vi "n3.vi"(6 "Analysis":u8, 7 "beta":dbl, 8 "m":dbl, 9 "P":dbl, 10 "Segmentation A":dbl[](array[numeric]), 11 "Segmentation B":dbl[](array[numeric])) -> (1 "X2_tau":dbl[][](array[numeric]), 2 "X2_i":dbl[][](array[numeric]))   [LabVIEW 2015]
uses:
  <vilib>/Analysis/baseanly.llb/Mean (DBL).vi
  <vilib>/Analysis/NI_AALBase.lvlib
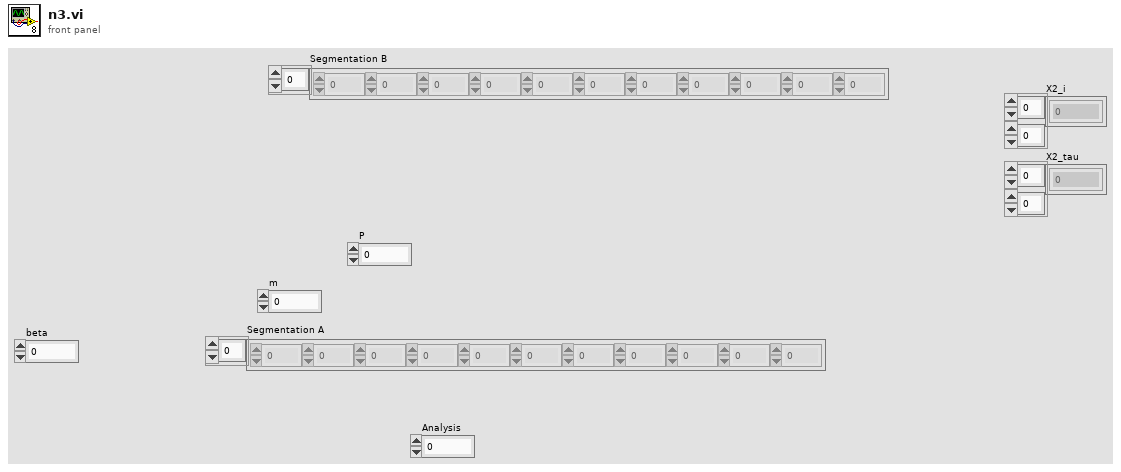
[diagram p1: front panel]
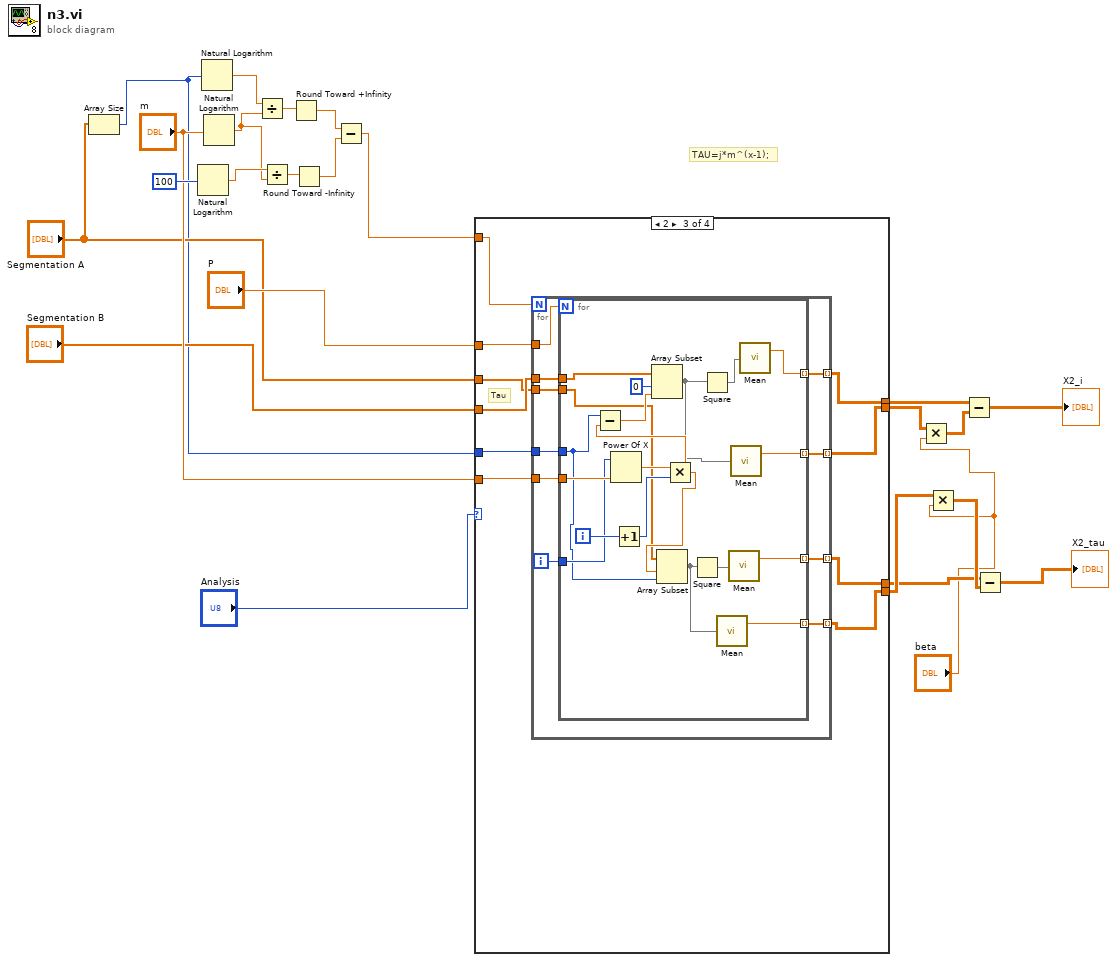
[diagram p0: block diagram]
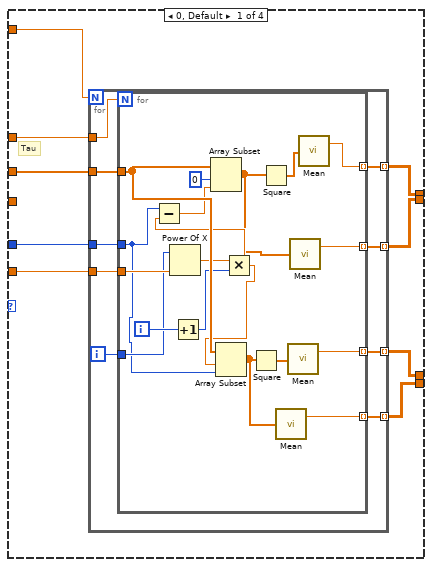
[diagram p2: hidden frame]
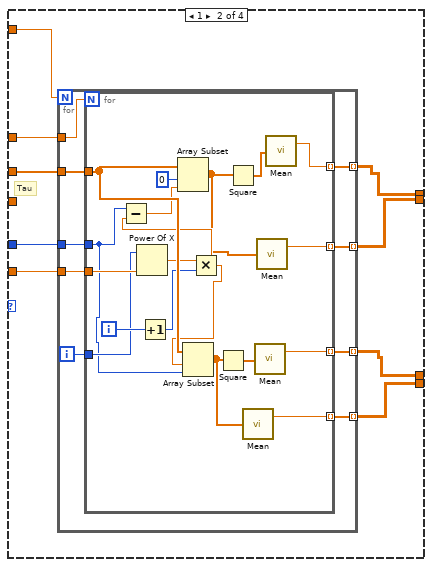
[diagram p3: hidden frame]
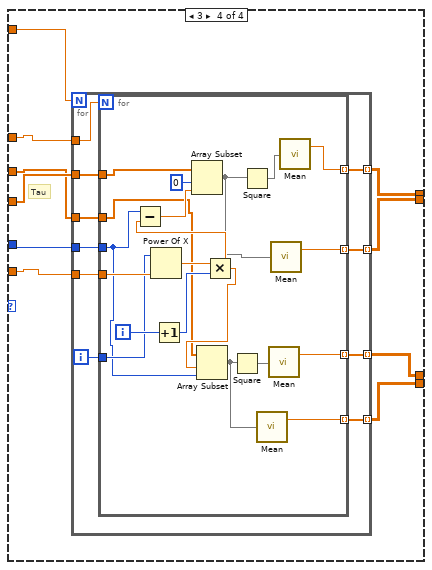
[diagram p4: hidden frame]
diagram:
  # "TAU=j*m^(x-1);"
  n1 = Array Size(array="Segmentation A") -> (size(s)=w4:i32)
  n2 = Natural Logarithm(1:100) -> (0:w21:dbl)
  n3 = Natural Logarithm(1:w4) -> (0:w24:dbl)
  n4 = Natural Logarithm(1:"m") -> (0:w20:dbl)
  n5 = Divide(x=w24, y=w20) -> (x/y=w23:dbl)
  n6 = Divide(x=w21, y=w20) -> (x/y=w18:dbl)
  n7 = Round Toward +Infinity(x=w23) -> (ceil(x): smallest int >= x=w19:dbl)
  n8 = Round Toward -Infinity(1:w18) -> (0:w17:dbl)
  n9 = Subtract(x=w19, y=w17) -> (x-y=w16:dbl)
  n10 = case shown="2" "Analysis" {
    tunnel: "Segmentation A" -> [w27 w69 w101 w136]
    tunnel: w4 -> [w26 w68 w104 w139]
    tunnel: w16 -> [w28 w67 w106 w140]
    tunnel: "m" -> [w25 w66 w103 w138]
    tunnel: "P" -> [w29 w65 w105 w141]
    tunnel: [w33 w64 w100 w142] -> w7
    tunnel: [w32 w63 w99 w143] -> w11
    tunnel: [w31 w62 w98 w144] -> w6
    tunnel: [w30 w61 w97 w145] -> w9
    tunnel: "Segmentation B" -> [_ _ w102 w137]
    frame 0, Default {
      # "Tau"
      n11 = for {
        N: w28 -> [_]
        tunnel: w29 -> [w42]
        tunnel: w27 -> [w41]
        tunnel: w26 -> [w40]
        tunnel: w25 -> [w39]
        tunnel: [w38] -> w33 mode=indexing
        tunnel: [w37] -> w32 mode=indexing
        tunnel: [w35] -> w31 mode=indexing
        tunnel: [w34] -> w30 mode=indexing
        i -> [w36]
        n12 = for {
          N: w42 -> [_]
          tunnel: w41 -> [w57]
          tunnel: w40 -> [w49]
          tunnel: w39 -> [w60]
          tunnel: w36 -> [w51]
          tunnel: [w59] -> w38 mode=indexing
          tunnel: [w58] -> w37 mode=indexing
          tunnel: [w55] -> w35 mode=indexing
          tunnel: [w54] -> w34 mode=indexing
          i -> [w53]
          n13 = Power Of X(1:w60, 2:w51) -> (0:w43:dbl)
          n14 = Increment(x=w53) -> (x+1=w52:i32)
          n15 = Multiply(x=w43, y=w52) -> (x*y=w50:dbl)
          n16 = Subtract(x=w49, y=w50) -> (x-y=w47:dbl)
          n17 = Array Subset(array=w57, index=0, length=w47) -> (w48:dbl[])
          n18 = Array Subset(array=w57, index=w50, length=w49) -> (w44:dbl[])
          n19 = Square(x=w44) -> (x^2=w56:dbl[])
          n20 = Square(x=w48) -> (x^2=w45:dbl[])
          n21 = call-poly <vilib>:"Mean.vi"("X"=w44) -> ("mean"=w54:dbl)  [unwired: 1 out]
          n22 = call-poly <vilib>:"Mean.vi"("X"=w56) -> ("mean"=w55:dbl)  [unwired: 1 out]
          n23 = call-poly <vilib>:"Mean.vi"("X"=w48) -> ("mean"=w58:dbl)  [unwired: 1 out]
          n24 = call-poly <vilib>:"Mean.vi"("X"=w45) -> ("mean"=w59:dbl)  [unwired: 1 out]
        }
      }
    }
    frame 1 {
      # "Tau"
      n25 = for {
        N: w67 -> [_]
        tunnel: w65 -> [w78]
        tunnel: w69 -> [w77]
        tunnel: w68 -> [w76]
        tunnel: w66 -> [w75]
        tunnel: [w74] -> w64 mode=indexing
        tunnel: [w73] -> w63 mode=indexing
        tunnel: [w71] -> w62 mode=indexing
        tunnel: [w70] -> w61 mode=indexing
        i -> [w72]
        n26 = for {
          N: w78 -> [_]
          tunnel: w77 -> [w93]
          tunnel: w76 -> [w83]
          tunnel: w75 -> [w96]
          tunnel: w72 -> [w86]
          tunnel: [w95] -> w74 mode=indexing
          tunnel: [w94] -> w73 mode=indexing
          tunnel: [w91] -> w71 mode=indexing
          tunnel: [w89] -> w70 mode=indexing
          i -> [w88]
          n27 = Power Of X(1:w96, 2:w86) -> (0:w85:dbl)
          n28 = Increment(x=w88) -> (x+1=w87:i32)
          n29 = Multiply(x=w85, y=w87) -> (x*y=w84:dbl)
          n30 = Subtract(x=w83, y=w84) -> (x-y=w81:dbl)
          n31 = Array Subset(array=w93, index=0, length=w81) -> (w82:dbl[])
          n32 = Array Subset(array=w93, index=w84, length=w83) -> (w90:dbl[])
          n33 = Square(x=w90) -> (x^2=w92:dbl[])
          n34 = Square(x=w82) -> (x^2=w79:dbl[])
          n35 = call-poly <vilib>:"Mean.vi"("X"=w90) -> ("mean"=w89:dbl)  [unwired: 1 out]
          n36 = call-poly <vilib>:"Mean.vi"("X"=w92) -> ("mean"=w91:dbl)  [unwired: 1 out]
          n37 = call-poly <vilib>:"Mean.vi"("X"=w82) -> ("mean"=w94:dbl)  [unwired: 1 out]
          n38 = call-poly <vilib>:"Mean.vi"("X"=w79) -> ("mean"=w95:dbl)  [unwired: 1 out]
        }
      }
    }
    frame 2 {
      # "Tau"
      n39 = for {
        N: w106 -> [_]
        tunnel: w105 -> [w116]
        tunnel: w102 -> [w115]
        tunnel: w104 -> [w114]
        tunnel: w103 -> [w113]
        tunnel: [w112] -> w100 mode=indexing
        tunnel: [w111] -> w99 mode=indexing
        tunnel: [w109] -> w98 mode=indexing
        tunnel: [w108] -> w97 mode=indexing
        tunnel: w101 -> [w107]
        i -> [w110]
        n40 = for {
          N: w116 -> [_]
          tunnel: w115 -> [w118]
          tunnel: w114 -> [w123]
          tunnel: w113 -> [w135]
          tunnel: w110 -> [w126]
          tunnel: [w134] -> w112 mode=indexing
          tunnel: [w133] -> w111 mode=indexing
          tunnel: [w131] -> w109 mode=indexing
          tunnel: [w129] -> w108 mode=indexing
          tunnel: w107 -> [w117]
          i -> [w128]
          n41 = Power Of X(1:w135, 2:w126) -> (0:w125:dbl)
          n42 = Increment(x=w128) -> (x+1=w127:i32)
          n43 = Multiply(x=w125, y=w127) -> (x*y=w124:dbl)
          n44 = Subtract(x=w123, y=w124) -> (x-y=w121:dbl)
          n45 = Array Subset(array=w118, index=0, length=w121) -> (w122:dbl[])
          n46 = Array Subset(array=w117, index=w124, length=w123) -> (w130:dbl[])
          n47 = Square(x=w130) -> (x^2=w132:dbl[])
          n48 = Square(x=w122) -> (x^2=w119:dbl[])
          n49 = call-poly <vilib>:"Mean.vi"("X"=w130) -> ("mean"=w129:dbl)  [unwired: 1 out]
          n50 = call-poly <vilib>:"Mean.vi"("X"=w132) -> ("mean"=w131:dbl)  [unwired: 1 out]
          n51 = call-poly <vilib>:"Mean.vi"("X"=w122) -> ("mean"=w133:dbl)  [unwired: 1 out]
          n52 = call-poly <vilib>:"Mean.vi"("X"=w119) -> ("mean"=w134:dbl)  [unwired: 1 out]
        }
      }
    }
    frame 3 {
      # "Tau"
      n53 = for {
        N: w140 -> [_]
        tunnel: w141 -> [w155]
        tunnel: w137 -> [w154]
        tunnel: w139 -> [w153]
        tunnel: w138 -> [w152]
        tunnel: [w151] -> w142 mode=indexing
        tunnel: [w150] -> w143 mode=indexing
        tunnel: [w148] -> w144 mode=indexing
        tunnel: [w147] -> w145 mode=indexing
        tunnel: w136 -> [w146]
        i -> [w149]
        n54 = for {
          N: w155 -> [_]
          tunnel: w154 -> [w171]
          tunnel: w153 -> [w161]
          tunnel: w152 -> [w174]
          tunnel: w149 -> [w164]
          tunnel: [w173] -> w151 mode=indexing
          tunnel: [w172] -> w150 mode=indexing
          tunnel: [w169] -> w148 mode=indexing
          tunnel: [w167] -> w147 mode=indexing
          tunnel: w146 -> [w156]
          i -> [w166]
          n55 = Power Of X(1:w174, 2:w164) -> (0:w163:dbl)
          n56 = Increment(x=w166) -> (x+1=w165:i32)
          n57 = Multiply(x=w163, y=w165) -> (x*y=w162:dbl)
          n58 = Subtract(x=w161, y=w162) -> (x-y=w159:dbl)
          n59 = Array Subset(array=w171, index=0, length=w159) -> (w160:dbl[])
          n60 = Array Subset(array=w156, index=w162, length=w161) -> (w168:dbl[])
          n61 = Square(x=w168) -> (x^2=w170:dbl[])
          n62 = Square(x=w160) -> (x^2=w157:dbl[])
          n63 = call-poly <vilib>:"Mean.vi"("X"=w168) -> ("mean"=w167:dbl)  [unwired: 1 out]
          n64 = call-poly <vilib>:"Mean.vi"("X"=w170) -> ("mean"=w169:dbl)  [unwired: 1 out]
          n65 = call-poly <vilib>:"Mean.vi"("X"=w160) -> ("mean"=w172:dbl)  [unwired: 1 out]
          n66 = call-poly <vilib>:"Mean.vi"("X"=w157) -> ("mean"=w173:dbl)  [unwired: 1 out]
        }
      }
    }
  }
  n67 = Multiply(x=w11, y="beta") -> (x*y=w10:dbl[][])
  n68 = Multiply(x=w9, y="beta") -> (x*y=w8:dbl[][])
  n69 = Subtract(x=w7, y=w10) -> (x-y=→"X2_i":dbl[][])
  n70 = Subtract(x=w6, y=w8) -> (x-y=→"X2_tau":dbl[][])
